vi "RSA Sign Hash.vi"(7 "private_key":string, 8 "error in (no error)":errorcluster, 10 "data":u8[](array[numeric]), 11 "RSA in":refnum<class "RSA.lvclass">) -> (0 "error out":errorcluster, 2 "signed_data":u8[](array[numeric]), 3 "RSA out":refnum<class "RSA.lvclass">)   [LabVIEW 2021, in "RSA.lvclass"]
uses:
  RSA.lvclass
  RSA.lvclass/RSA.ctl
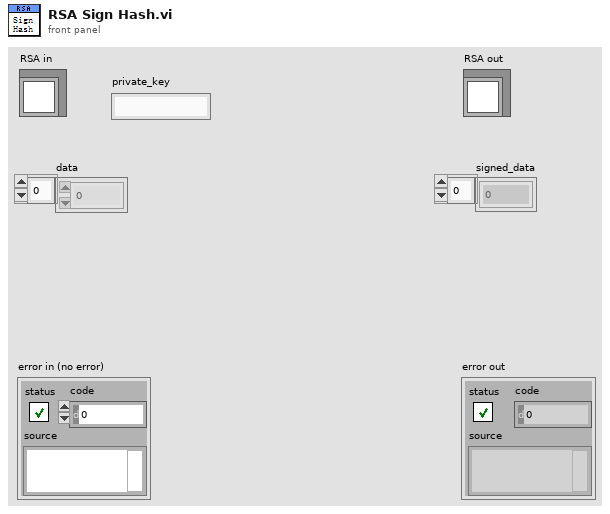
[diagram p1: front panel]
types:
  T1 = enum16{"MD5", "SHA1", "SHA256", "SHA384", "SHA512"}
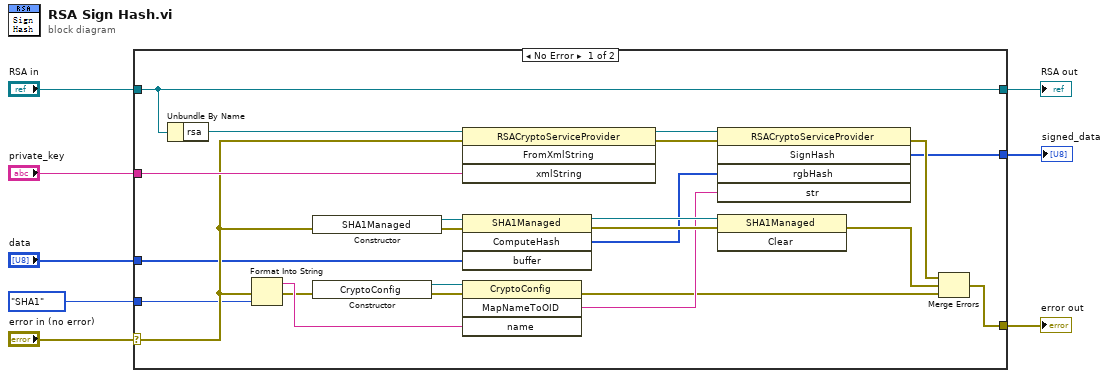
[diagram p0: block diagram]
diagram:
  n1 = case shown="No Error" "error in (no error)" {
    selector: "error in (no error)" -> [w21 w33]
    tunnel: [w14 w33] -> w7
    tunnel: [w28 w32] -> w5
    tunnel: "RSA in" -> [w28 w32]
    tunnel: "private_key" -> [w31 _]
    tunnel: T1."SHA1" ("oid_type") -> [w20 _]
    tunnel: [w13 _] -> w2
    tunnel: "data" -> [w9 _]
    frame No Error {
      n2 = Unbundle By Name(w28) -> ("rsa"=w27:refnum<k24>)
      n3 = Format Into String(error in=w21, w20) -> (resulting string=w18:string, error out=w12:errorcluster)  [unwired: 2 in]
      n4 = constructor class="SHA1Managed" ("AliceEntschlüsselt")(error in=w21) -> (reference out=w23:refnum<k24>, error out=w24:errorcluster)  [unwired: 2 in, 1 out]
      n5 = constructor class="CryptoConfig" ("AliceEntschlüsselt")(error in=w12) -> (reference out=w10:refnum<k24>, error out=w11:errorcluster)  [unwired: 2 in, 1 out]
      n6 = invoke class="RSACryptoServiceProvider" method="FromXmlString"(reference=w27, error in=w21, "xmlString"=w31) -> (reference out=w29:refnum<k24>, error out=w30:errorcluster)  [unwired: 1 in, 2 out]
      n7 = invoke class="SHA1Managed" method="ComputeHash"(reference=w23, error in=w24, "buffer"=w9) -> (reference out=w26:refnum<k24>, error out=w25:errorcluster, "ComputeHash"=w22:u8[])  [unwired: 1 in, 1 out]
      n8 = invoke class="CryptoConfig" method="MapNameToOID"(reference=w10, error in=w11, "name"=w18) -> (error out=w17:errorcluster, "MapNameToOID"=w19:string)  [unwired: 1 in, 2 out]
      n9 = invoke class="RSACryptoServiceProvider" method="SignHash"(reference=w29, error in=w30, "rgbHash"=w22, "str"=w19) -> (error out=w15:errorcluster, "SignHash"=w13:u8[])  [unwired: 1 in, 3 out]
      n10 = invoke class="SHA1Managed" method="Clear"(reference=w26, error in=w25) -> (error out=w16:errorcluster)  [unwired: 1 in, 2 out]
      n11 = Merge Errors(w15, w16, w17) -> (w14:errorcluster)
    }
    frame Error {
    }
  }
  "error out" <- w7
  "RSA out" <- w5
  "signed_data" <- w2
